vi "is Result Ready.vi"(8 "error in (no error)":errorcluster, 11 "Cap Bank Idot Measurement in":refnum<class "Cap Bank Idot Measurement.lvclass">) -> (0 "error out":errorcluster, 2 "Result Available":bool=TRUE, 3 "Cap Bank Idot Measurement out":refnum<class "Cap Bank Idot Measurement.lvclass">)   [LabVIEW 2015, in "Cap Bank Idot Measurement.lvclass"]
uses:
  Cap Bank Idot Measurement.lvclass
  NI-DAQ/Mag Lab Measure/DAQmx Digitizer/DAQmx Digitizer.lvclass
  Mag Lab Error Handler/Mag Lab Error Handler.lvclass
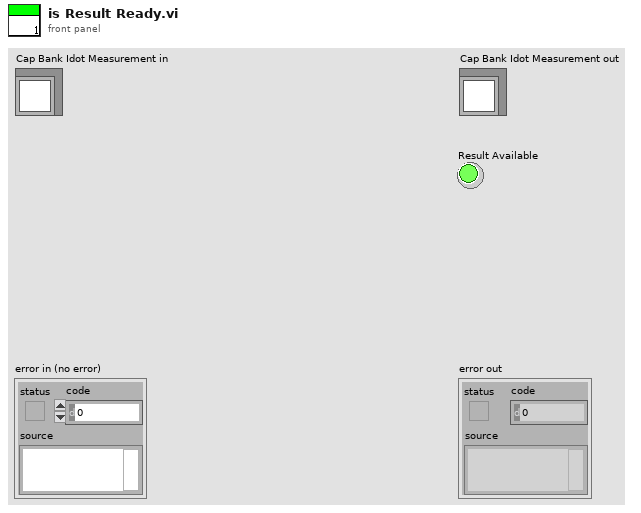
[diagram p1: front panel]
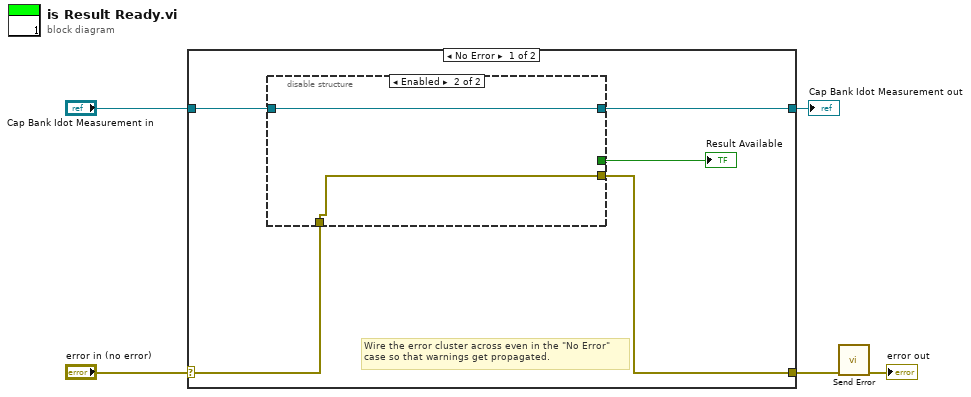
[diagram p0: block diagram]
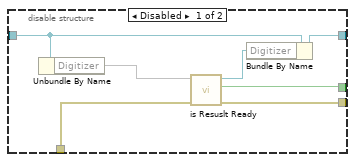
[diagram p2: hidden frame]
diagram:
  n1 = case shown="No Error" "error in (no error)" {
    selector: "error in (no error)" -> [w9 w21]
    tunnel: [w8 w21] -> w2
    tunnel: [w7 w20] -> w3
    tunnel: "Cap Bank Idot Measurement in" -> [w10 w20]
    frame No Error {
      # "Wire the error cluster across even in the \"No Error\"\ncase so that warnings get propagated."
      n2 = disable-structure shown="Enabled" {
        disable-tunnel: w10 -> [w17 w19]
        disable-tunnel: w9 -> [w15 w18]
        disable-tunnel: [w14 w18] -> w8
        disable-tunnel: [w13 w19] -> w7
        disable-tunnel: [w11 _] -> w6
        frame Disabled {
          n3 = Unbundle By Name(w17) -> ("Digitizer"=w16)
          n4 = call-dynamic "is Resuslt Ready.vi"("error in (no error)"=w15, "DAQmx Digitizer in"=w16) -> ("error out"=w14:errorcluster, "Result Available"=w11:bool, "DAQmx Digitizer out"=w12:refnum<class "DAQmx Digitizer.lvclass">)  [unwired: 7 in]
          n5 = Bundle By Name(cluster=w17, "Digitizer"=w12) -> (w13:refnum<class "Cap Bank Idot Measurement.lvclass">)
        }
        frame Enabled {
        }
      }
      "Result Available" <- w6
    }
    frame Error {
    }
  }
  "Cap Bank Idot Measurement out" <- w3
  n6 = call "Send Error.vi"("error in (no error)"=w2) -> ("error out"=→"error out":errorcluster)  [unwired: 9 in, 1 out]
